vi "AddFailure.vi"(7 "Time":dbl, 8 "error in (no error)":errorcluster, 9 "Failure":errorcluster, 10 "Test":refnum<class "Test.lvclass">, 11 "ResultTreeListener in":refnum<class "ResultTreeListener.lvclass">) -> (0 "error out":errorcluster, 3 "ResultTreeListener out":refnum<class "ResultTreeListener.lvclass">)   [LabVIEW 2019, in "ResultTreeListener.lvclass"]
doc: "A failure occurred."
uses:
  ResultTreeListener.lvclass
  Test/Test.lvclass
  ResultTreeListener.lvclass/ResultTreeListener.ctl
  ResultTree/ResultTree.lvclass
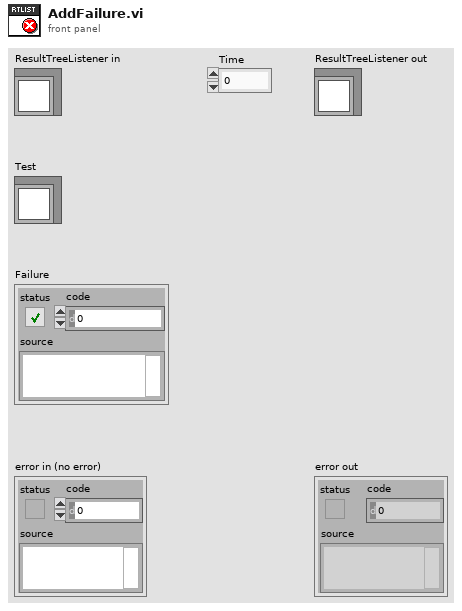
[diagram p1: front panel]
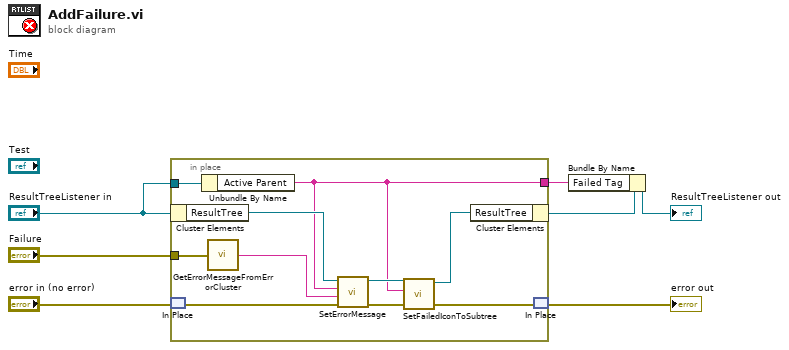
[diagram p0: block diagram]
diagram:
  n1 = in-place {
    in-place-border: "ResultTreeListener in" -> [w17]
    in-place-border: "Failure" -> [w15]
    in-place-border: [w8] -> w1
    n2 = in-place-cluster #1("ResultTreeListener in") -> ("ResultTree"=w12:refnum<class "ResultTree.lvclass">)
    n3 = in-place-match #2("error in (no error)") -> (w9:errorcluster)
    n4 = Unbundle By Name(w17) -> ("Active Parent"=w8:string)
    n5 = call "GetErrorMessageFromErrorCluster.vi"("error in (no error)"=w15) -> ("trimmed string"=w16:string)
    n6 = call "SetErrorMessage.vi"("error in (no error)"=w9, "Error Message"=w16, "Tag Name"=w8, "ResultTree in"=w12) -> ("error out"=w10:errorcluster, "ResultTree out"=w11:refnum<class "ResultTree.lvclass">)  [unwired: 6 in]
    n7 = call "SetFailedIconToSubtree.vi"("error in (no error)"=w10, "Active Parent"=w8, "ResultTree in"=w11) -> ("error out"=w14:errorcluster, "ResultTree out"=w13:refnum<class "ResultTree.lvclass">)  [unwired: 7 in]
    n8 = in-place-cluster #1("ResultTree"=w13) -> (w3:refnum<class "ResultTreeListener.lvclass">)
    n9 = in-place-match #2(w14) -> (→"error out":errorcluster)
  }
  n10 = Bundle By Name(cluster=w3, "Failed Tag"=w1) -> (→"ResultTreeListener out":refnum<class "ResultTreeListener.lvclass">)
